vi "select_config subVI.vi"(8 "error in (no error)":errorcluster, 10 "Power Supply Settings IN":T1, 11 "Configuration Standard":u16(ring) items=["UL", "IEC", "CHINA"]) -> (0 "error out":errorcluster, 3 "Power Supply Settings":T1)   [LabVIEW 2016]
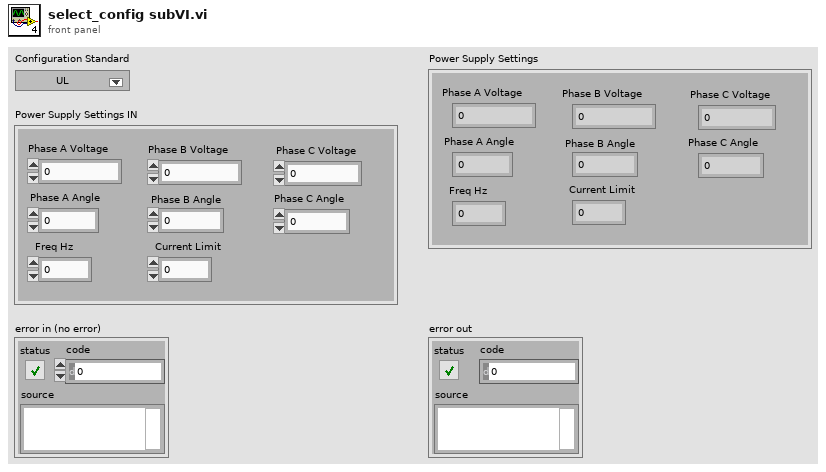
[diagram p1: front panel]
types:
  T1 = cluster{"Phase A Voltage":i32, "Phase B Voltage":i32, "Phase C Voltage":i32, "Phase A Angle":i32, "Phase B Angle":i32, "Phase C Angle":i32, "Freq Hz":i32, "Current Limit":i32}
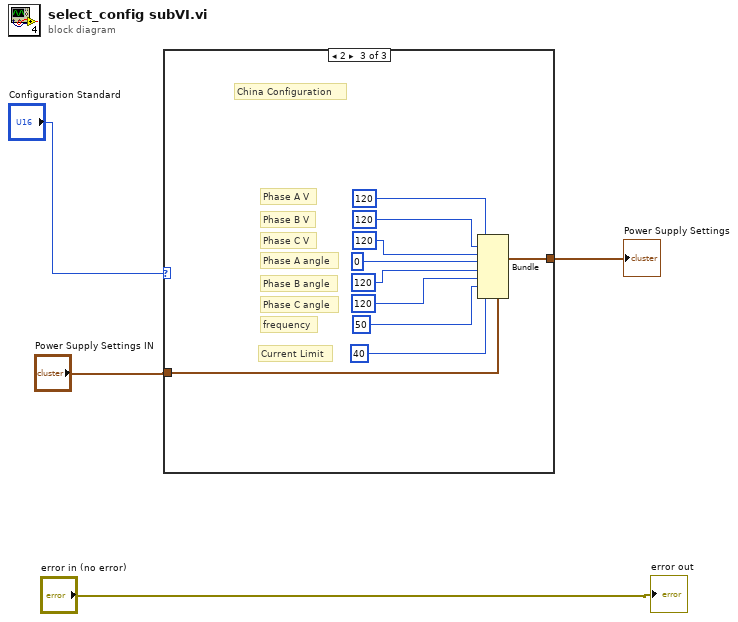
[diagram p0: block diagram]
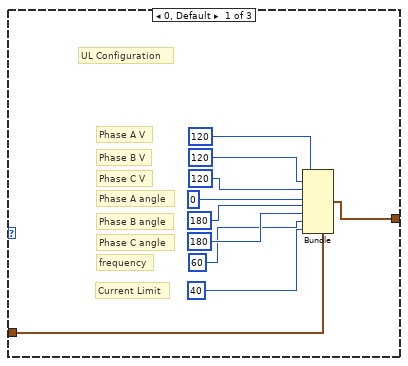
[diagram p2: hidden frame]
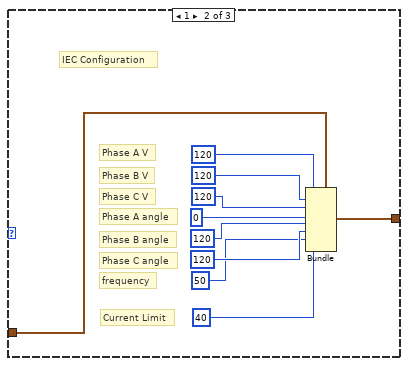
[diagram p3: hidden frame]
diagram:
  n1 = case shown="2" "Configuration Standard" {
    tunnel: "Power Supply Settings IN" -> [w6 w17 w26]
    tunnel: [w7 w16 w27] -> w3
    frame 0, Default {
      # "Current Limit"
      # "frequency"
      # "Phase C angle"
      # "Phase B angle"
      # "Phase A angle"
      # "Phase C V"
      # "Phase B V"
      # "Phase A V"
      # "UL Configuration"
      n2 = Bundle(cluster=w6, "Phase A Voltage"=120, "Phase B Voltage"=120, "Phase C Voltage"=120, "Phase A Angle"=0, "Phase B Angle"=180, "Phase C Angle"=180, "Freq Hz"=60, "Current Limit"=40) -> (w7:T1)
    }
    frame 1 {
      # "Current Limit"
      # "frequency"
      # "Phase C angle"
      # "Phase B angle"
      # "Phase A angle"
      # "Phase C V"
      # "Phase B V"
      # "Phase A V"
      # "IEC Configuration"
      n3 = Bundle(cluster=w17, "Phase A Voltage"=120, "Phase B Voltage"=120, "Phase C Voltage"=120, "Phase A Angle"=0, "Phase B Angle"=120, "Phase C Angle"=120, "Freq Hz"=50, "Current Limit"=40) -> (w16:T1)
    }
    frame 2 {
      # "Current Limit"
      # "frequency"
      # "Phase C angle"
      # "Phase B angle"
      # "Phase A angle"
      # "Phase C V"
      # "Phase B V"
      # "Phase A V"
      # "China Configuration"
      n4 = Bundle(cluster=w26, "Phase A Voltage"=120, "Phase B Voltage"=120, "Phase C Voltage"=120, "Phase A Angle"=0, "Phase B Angle"=120, "Phase C Angle"=120, "Freq Hz"=50, "Current Limit"=40) -> (w27:T1)
    }
  }
  "Power Supply Settings" <- w3
  "error out" <- "error in (no error)"
